vi "Helmholtz2D_Cal Coef Mtrx_Neumann.vi"(9 "Domain":T2={"x"={"start x"=0.0, "end x"=1.0, "# of x-points"=11}, "y"={"start y"=0.0, "end y"=1.0, "# of y-points"=11}}, 10 "a":dbl, 11 "k":dbl=1.0) -> (2 "D":T1, 3 "C":T1)   [LabVIEW 2020, in "NI_PDE.lvlib"]
uses:
  <vilib>/gmath/NI_PDE.lvlib
  <vilib>/Analysis/Matrix/Datatypes/RealMatrix.ctl
  <vilib>/Analysis/7linalg.llb/Create Special Real Matrix.vi
  <vilib>/Analysis/Matrix/Numeric/Multiply/Multiply - R,RM.vi
  <vilib>/Analysis/Matrix/Numeric/Multiply/Multiply - RM,R.vi
  <vilib>/Analysis/Matrix/Numeric/Add/Add - RM,RM.vi
  <vilib>/Analysis/NI_AALPro.lvlib
  <vilib>/Analysis/Matrix/NI_Matrix.lvlib
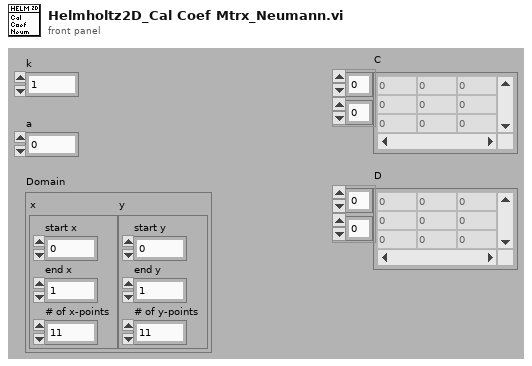
[diagram p1: front panel]
types:
  T1 = typedef "NI_Matrix.lvlib/RealMatrix.ctl" = dbl[][]
  T2 = cluster{"x":cluster{"start x":dbl, "end x":dbl, "# of x-points":i32}, "y":cluster{"start y":dbl, "end y":dbl, "# of y-points":i32}}
  T3 = enum32{"Identity", "Diagonal", "Toepliz", "Vandermonde", "Companion"}
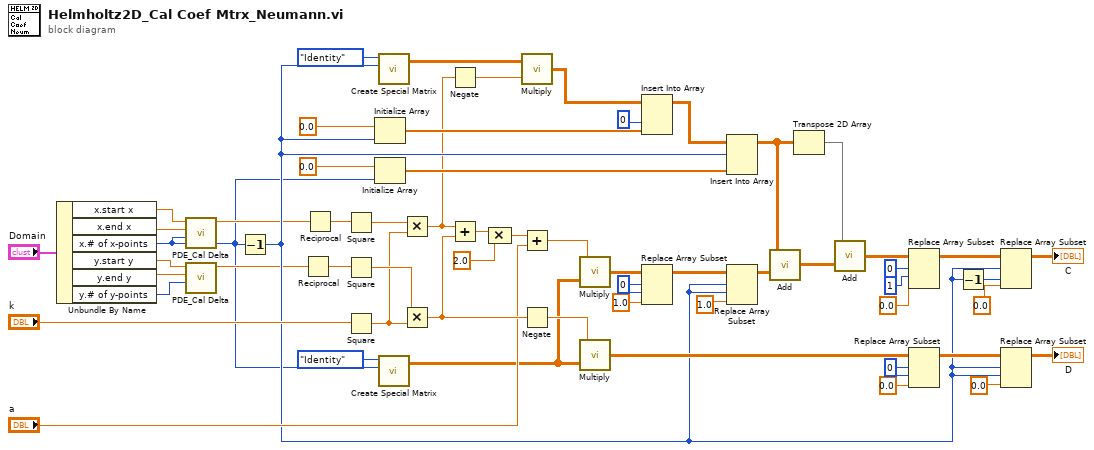
[diagram p0: block diagram]
diagram:
  w17 = 0 ("index (row)")
  w36 = 0 ("index (row)")
  n1 = Unbundle By Name("Domain") -> ("x.start x"=w59:dbl, "x.end x"=w58:dbl, "x.# of x-points"=w3:i32, "y.start y"=w56:dbl, "y.end y"=w57:dbl, "y.# of y-points"=w55:i32)
  n2 = call <vilib>:"PDE_Cal Delta.vi"("# of points"=w3, "end"=w58, "start"=w59) -> ("delta"=w6:dbl)  [unwired: 8 out]
  n3 = call <vilib>:"PDE_Cal Delta.vi"("# of points"=w55, "end"=w57, "start"=w56) -> ("delta"=w7:dbl)  [unwired: 8 out]
  n4 = Decrement(x=w3) -> (x-1=w10:i32)
  n5 = Reciprocal(x=w7) -> (1/x=w1:dbl)
  n6 = Reciprocal(x=w6) -> (1/x=w2:dbl)
  n7 = Square(x=w2) -> (x^2=w24:dbl)
  n8 = Square(x=w1) -> (x^2=w25:dbl)
  n9 = Square(x="k") -> (x^2=w23:dbl)
  n10 = Initialize Array(0.0 ("element"), w10) -> (w47:dbl[])
  n11 = Initialize Array(0.0 ("element"), w3) -> (w43:dbl[])
  n12 = call-poly <vilib>:"Create Special Matrix.vi"("matrix type"=T3."Identity", "matrix size"=w10) -> ("Special Matrix"=w50:T1)  [unwired: 2 in, 2 out]
  n13 = call-poly <vilib>:"Create Special Matrix.vi"("matrix type"=T3."Identity", "matrix size"=w3) -> ("Special Matrix"=w8:T1)  [unwired: 2 in, 2 out]
  n14 = Multiply(x=w24, y=w23) -> (x*y=w9:dbl)
  n15 = Multiply(x=w25, y=w23) -> (x*y=w21:dbl)
  n16 = Negate(x=w9) -> (-x=w18:dbl)
  n17 = Add(x=w9, y=w21) -> (x+y=w52:dbl)
  n18 = Compound Arithmetic op=MULTIPLY(w52, 2.0 ("y")) -> (w26:dbl)
  n19 = call-poly <vilib>:"Multiply.vi"("Real Scalar c"=w18, "Real Matrix A"=w50) -> ("A * c"=w48:T1)
  n20 = Add(x=w26, y="a") -> (x+y=w20:dbl)
  n21 = Negate(x=w21) -> (-x=w19:dbl)
  n22 = call-poly <vilib>:"Multiply.vi"("Real Matrix A"=w8, "Real Scalar c"=w20) -> ("c * A"=w35:T1)
  n23 = call-poly <vilib>:"Multiply.vi"("Real Matrix A"=w8, "Real Scalar c"=w19) -> ("c * A"=w15:T1)
  n24 = Insert Into Array(array=w48, index (col)=0 ("disabled index (col)"), new element=w47) -> (w45:T1)  [unwired: 1 in]
  n25 = Replace Array Subset(array=w35, new element=1.0 ("new element/subarray"), index (row)=w36, index (col)=w36) -> (w38:T1)
  n26 = Insert Into Array(array=w45, index (row)=w10, new element=w43) -> (w42:T1)  [unwired: 1 in]
  n27 = Replace Array Subset(array=w38, new element=1.0 ("new element/subarray"), index (row)=w10, index (col)=w10) -> (w34:T1)
  n28 = call-poly <vilib>:"Add.vi"("Real Matrix B"=w34, "Real Matrix A"=w42) -> ("A + B"=w41:T1)
  n29 = Transpose 2D Array(2D array=w42) -> (transposed array=w40:T1)
  n30 = call-poly <vilib>:"Add.vi"("Real Matrix B"=w41, "Real Matrix A"=w40) -> ("A + B"=w30:T1)
  n31 = Replace Array Subset(array=w30, new element=0.0 ("new element/subarray"), index (row)=0, index (col)=1 ("index (row)")) -> (w33:T1)
  n32 = Replace Array Subset(array=w15, new element=0.0 ("new element/subarray"), index (row)=w17, index (col)=w17) -> (w13:T1)
  n33 = Decrement(x=w10) -> (x-1=w27:i32)
  n34 = Replace Array Subset(array=w33, new element=0.0 ("new element/subarray"), index (row)=w10, index (col)=w27) -> (→"C":T1)
  n35 = Replace Array Subset(array=w13, new element=0.0 ("new element/subarray"), index (row)=w10, index (col)=w10) -> (→"D":T1)
